vi "Authenticate with Access Token.vi"(5 "Base URL":string, 6 "Body Parameters":T4[](array[typedef]), 7 "HTTP Method":T5, 8 "error in (no error)":errorcluster, 9 "Header Parameters":T4[](array[typedef]), 10 "URL Parameters":T4[](array[typedef]), 11 "OAuth Handle":T1={"Signature Method"=enum."HMAC-SHA1", "Version"="", "Client"={"Token"="", "Secret"=""}, "Access"={"Token"="", "Secret"=""}}) -> (0 "error out":errorcluster, 1 "Header Value":string, 2 "Header Parameter":string, 3 "Full URL":string, 4 "Body":string)   [LabVIEW 2011, in "i3-oauth.lvlib"]
doc: "Creates the OAuth signature and Authorization Header for a HTTP request. The Authenticate with Access Token VI should be passed all parameters that the service requires to be signed as part of the request. \n\nUse the <b>Build Parameter VI</b> along with the standard Build Array VI in LabVIEW to create the arrays for the following types of parameters:\n\n<b>URL Parameters</b> that are provided are used as part of the signature and added to the <b>Base URL</B> (the service URL without URL parameters) in order to create the <b>Full URL</b> used for the HTTP Request.\n\n<b>Header Parameters</b> consist only of parameters that are part of the OAuth signature and should appear as part of the \"OAuth\" header element. The VI returns the <b>Header Parameter</b> and the <b>Header Value</b> that should be added to the HTTP Request. This VI <b>includes</b> the Client Credentials and the Access Credentials from the OAuth Handle. This VI should be used after an Authentication Workflow, such as the Browser Workflow Authentication, so the Access Credentials for the user are available.\n\n<b>Body Parameters</b> are parameters that the service expects to be part of the OAuth signature for the HTTP request. The <b>Body</b> return is an application/x-www-form-urlencoded version of the Body Parameters which is the encoding used by most web services for HTTP body data."
uses:
  i3-oauth.lvlib
  Controls/Name-Value Pair.ctl
  Controls/HTTP Method.ctl
  Controls/OAuth Handle.ctl
  Controls/Signature Method.ctl
  Controls/Credentials.ctl
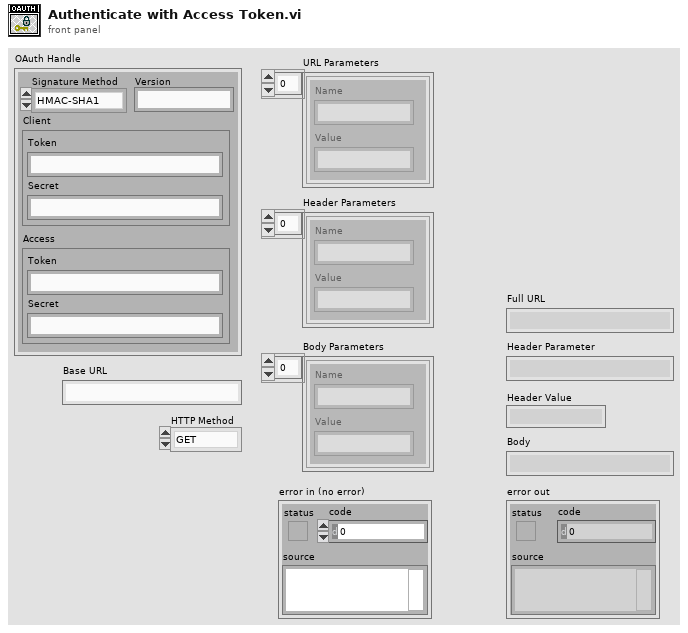
[diagram p1: front panel]
types:
  T1 = typedef "i3-oauth.lvlib/OAuth Handle.ctl" = cluster{"Signature Method":T2, "Version":string, "Client":T3, "Access":T3}
  T2 = typedef "i3-oauth.lvlib/Signature Method.ctl" = enum16{"HMAC-MD5", "HMAC-SHA1", "HMAC-SHA224", "HMAC-SHA256", "HMAC-SHA384", "HMAC-SHA512"}
  T3 = typedef "i3-oauth.lvlib/Credentials.ctl" = cluster{"Token":string, "Secret":string}
  T4 = typedef "i3-oauth.lvlib/Name-Value Pair.ctl" = cluster{"Name":string, "Value":string}
  T5 = typedef "i3-oauth.lvlib/HTTP Method.ctl" = enum16{"GET", "POST", "PUT", "DELETE"}
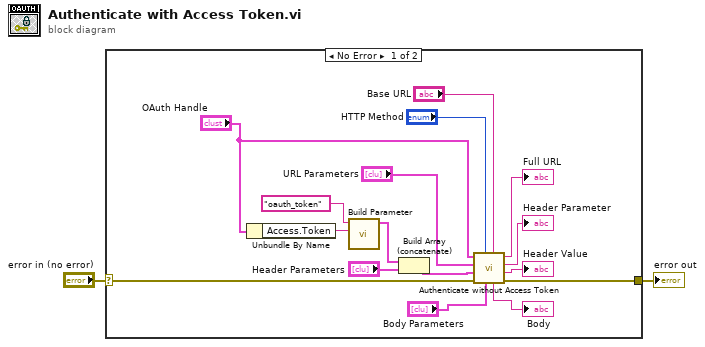
[diagram p0: block diagram]
diagram:
  n1 = case shown="No Error" "error in (no error)" {
    selector: "error in (no error)" -> [w14 w19]
    tunnel: [w15 w19] -> w2
    frame No Error {
      n2 = Unbundle By Name("OAuth Handle") -> ("Access.Token"=w10:string)
      n3 = call "Build Parameter.vi"("Value"=w10, "Key"="oauth_token") -> ("Parameter Array"=w6:T4[])  [unwired: 9 in]
      n4 = Build Array (concatenate)(w6, "Header Parameters") -> (w8:T4[])
      n5 = call "Authenticate without Access Token.vi"("Base URL"="Base URL", "Body Parameters"="Body Parameters", "HTTP Method"="HTTP Method", "error in (no error)"=w14, "Header Parameters"=w8, "URL Parameters"="URL Parameters", "OAuth Handle"="OAuth Handle") -> ("error out"=w15:errorcluster, "Header Value"=→"Header Value":string, "Header Parameter"=→"Header Parameter":string, "Full URL"=→"Full URL":string, "Body"=→"Body":string)
    }
    frame Error {
    }
  }
  "error out" <- w2
